vi "Get Instrument Type ID.vi"(8 "error in (no error)":errorcluster, 11 "session factory in":refnum<class "ISession Factory.lvclass">) -> (0 "error out":errorcluster, 2 "instrument type id":string, 3 "session factory out":refnum<class "ISession Factory.lvclass">)   [LabVIEW 2020, in "MeasurementLink Instrument.lvlib" / "ISession Factory.lvclass"]
doc: "Returns the type ID for the instrument in the pin map file. When using third party instruments not natively supported by the pin map editor, you must create a custom instrument in the pin map file and assign it a unique instrument type ID. Return the same instrument type ID from this method to access the third party instrument from within MeasurementLink."
uses:
  ISession Factory.lvclass
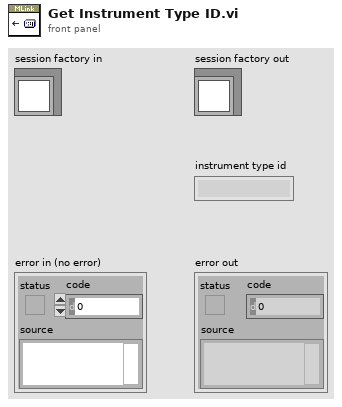
[diagram p1: front panel]
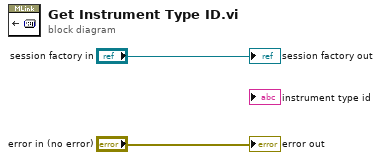
[diagram p0: block diagram]
diagram:
  "error out" <- "error in (no error)"
  "session factory out" <- "session factory in"
